vi "Kelvinox_Check_Queue.vi"(7 "error in (no error)":errorcluster, 10 "queue":refnum<queue>) -> (0 "error out":errorcluster, 1 "Kelvinox-Control":T1, 3 "New Entries?":bool)   [LabVIEW 2019]
uses:
  Kelvinox/Kelvinox_Control.ctl
panel:
  out "Numeric":i32
  # "Pressures in mbar"
  # "Temperatures in K"
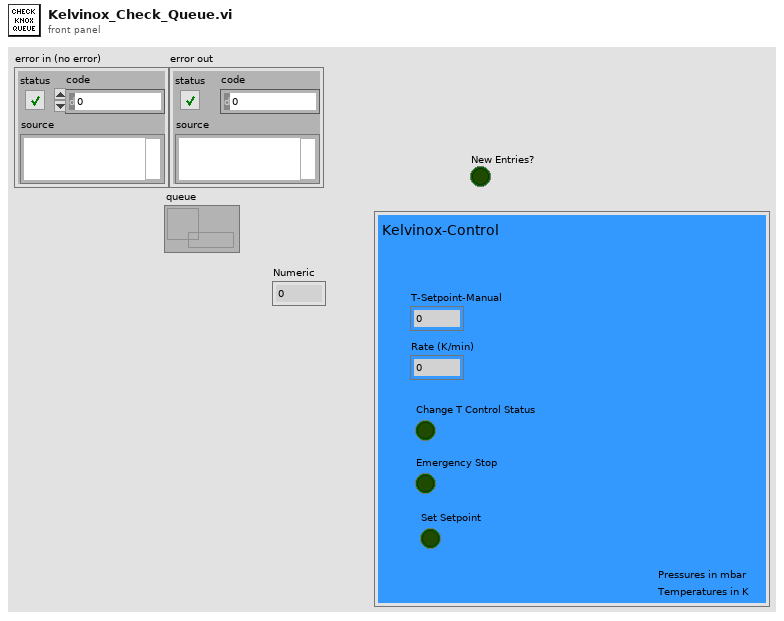
[diagram p1: front panel]
types:
  T1 = typedef "Kelvinox_Control.ctl" = cluster{"T-Setpoint-Manual":dbl, "Rate (K/min)":dbl, "Change T Control Status":bool, "Emergency Stop":bool, "Set Setpoint":bool}
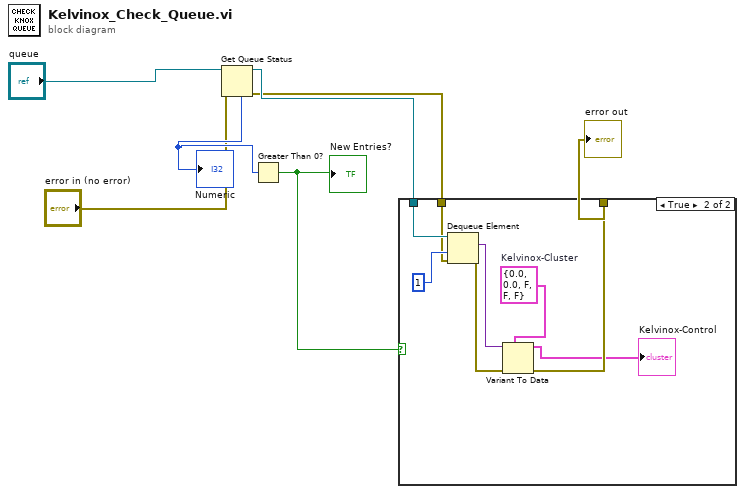
[diagram p0: block diagram]
diagram:
  n1 = Get Queue Status(queue="queue", error in (no error)="error in (no error)") -> (queue out=w6:refnum<queue>, error out=w4:errorcluster, # elements in queue=w7:i32)  [unwired: 1 in, 5 out]
  "Numeric" <- w7
  n2 = Greater Than 0?(x=w7) -> (x > 0?=w5:bool)
  "New Entries?" <- w5
  n3 = case shown="True" w5 {
    tunnel: w6 -> [_ w14]
    tunnel: w4 -> [w8 w13]
    tunnel: [w8 w11] -> w2
    frame False {
    }
    frame True {
      w9 = T1 {"T-Setpoint-Manual"=0.0, "Rate (K/min)"=0.0, "Change T Control Status"=FALSE, "Emergency Stop"=FALSE, "Set Setpoint"=FALSE}  # Kelvinox-Cluster
      n4 = Dequeue Element(queue=w14, timeout in ms (-1)=1, error in (no error)=w13) -> (element=w15:variant, error out=w12:errorcluster)  [unwired: 2 out]
      n5 = Variant To Data(error in=w12, type=w9, Variant=w15) -> (data=→"Kelvinox-Control":T1, error out=w11:errorcluster)
    }
  }
  "error out" <- w2
